vi "CCD spectrum processing_Shaowei-v5.vi"() -> ()   [LabVIEW 2012]
uses:
  <vilib>/Utility/file.llb/Read From Spreadsheet File (string).vi
  <vilib>/Utility/file.llb/Read From Spreadsheet File (DBL).vi
panel:
  out "Data Information":string[](array[string])
  in  "dI/dV Input Channel":i32=5
  out "File Information":string[][](array[string])
  out "Normalized dI/dV":cluster{"first row":dbl[], dbl[]}(graph)
  out "I":cluster{cluster{dbl, dbl}[]}[](graph)
  out "dI/dV":cluster{cluster{dbl, dbl}[]}[](graph)
  out "I":cluster{cluster{dbl, dbl}[]}[](graph)
  out "Spec1 File name 3":string
  out "Spec1 File name 2":string
  in  "select":bool
  in  "next":bool
  in  "previous":bool
  in  "Do it":bool
  out "?":path=path "F:/Bias-Spectroscopy113.dat"
  # "Input File"
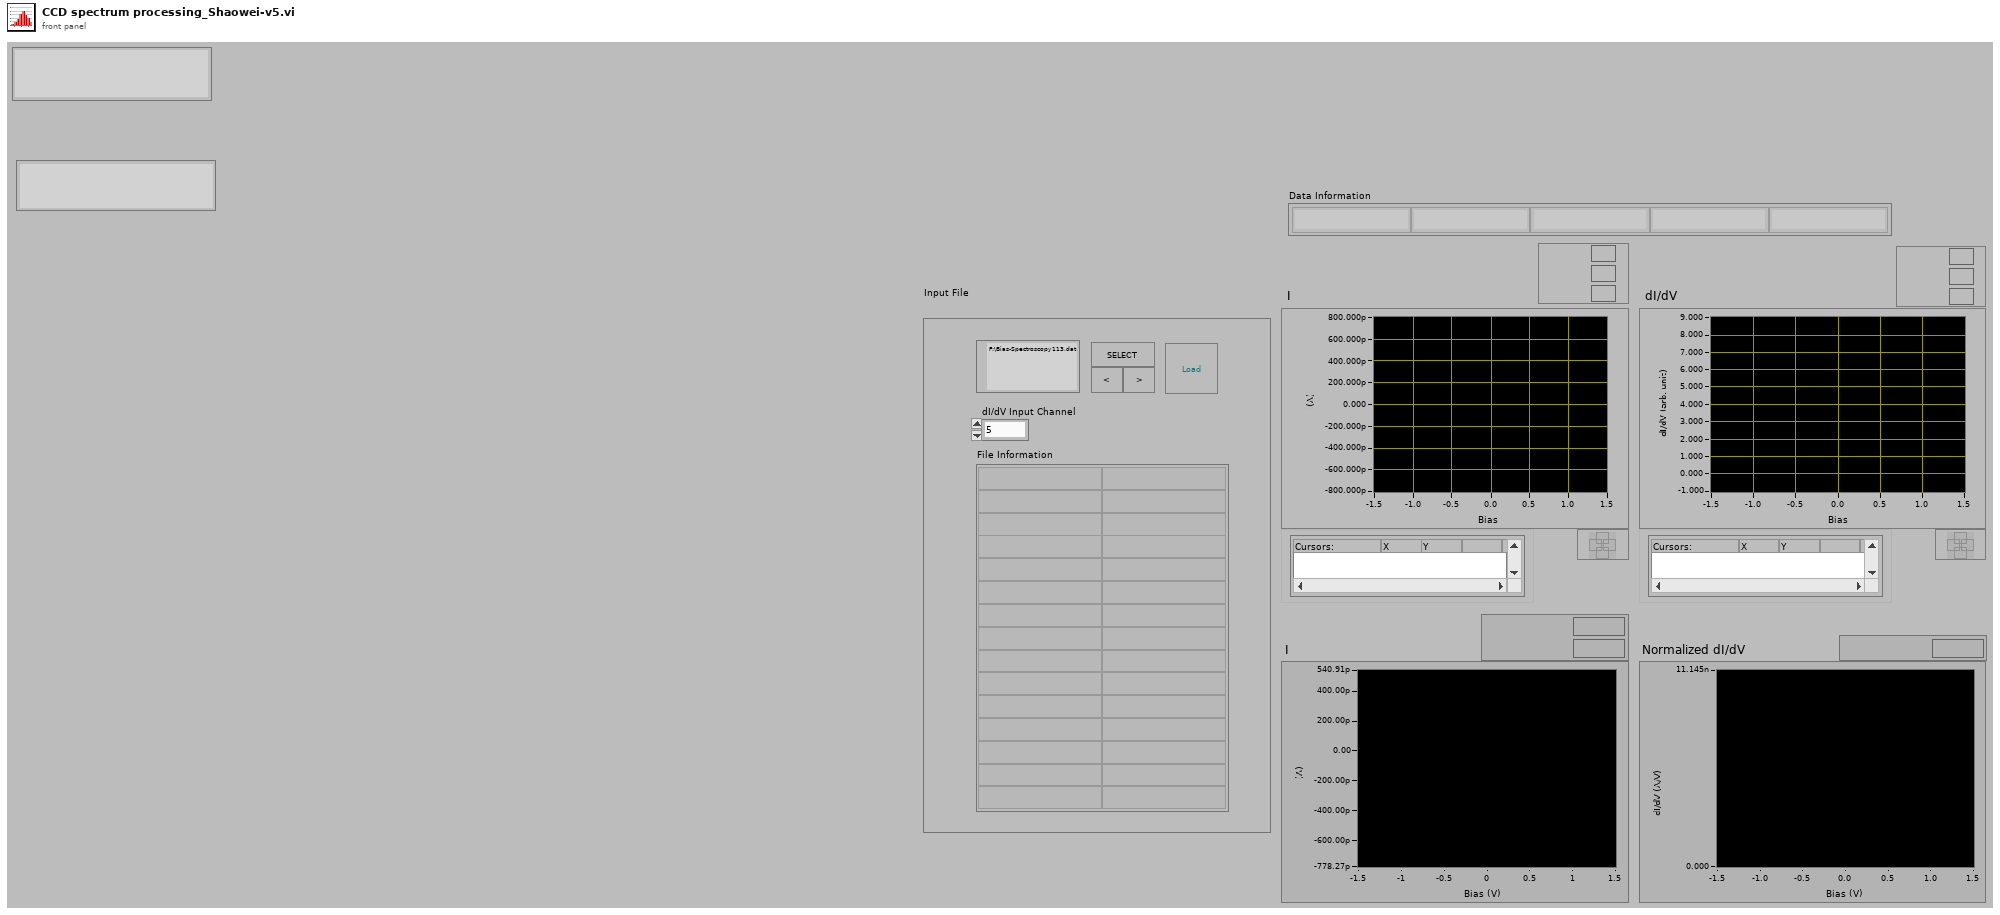
[diagram p1: front panel]
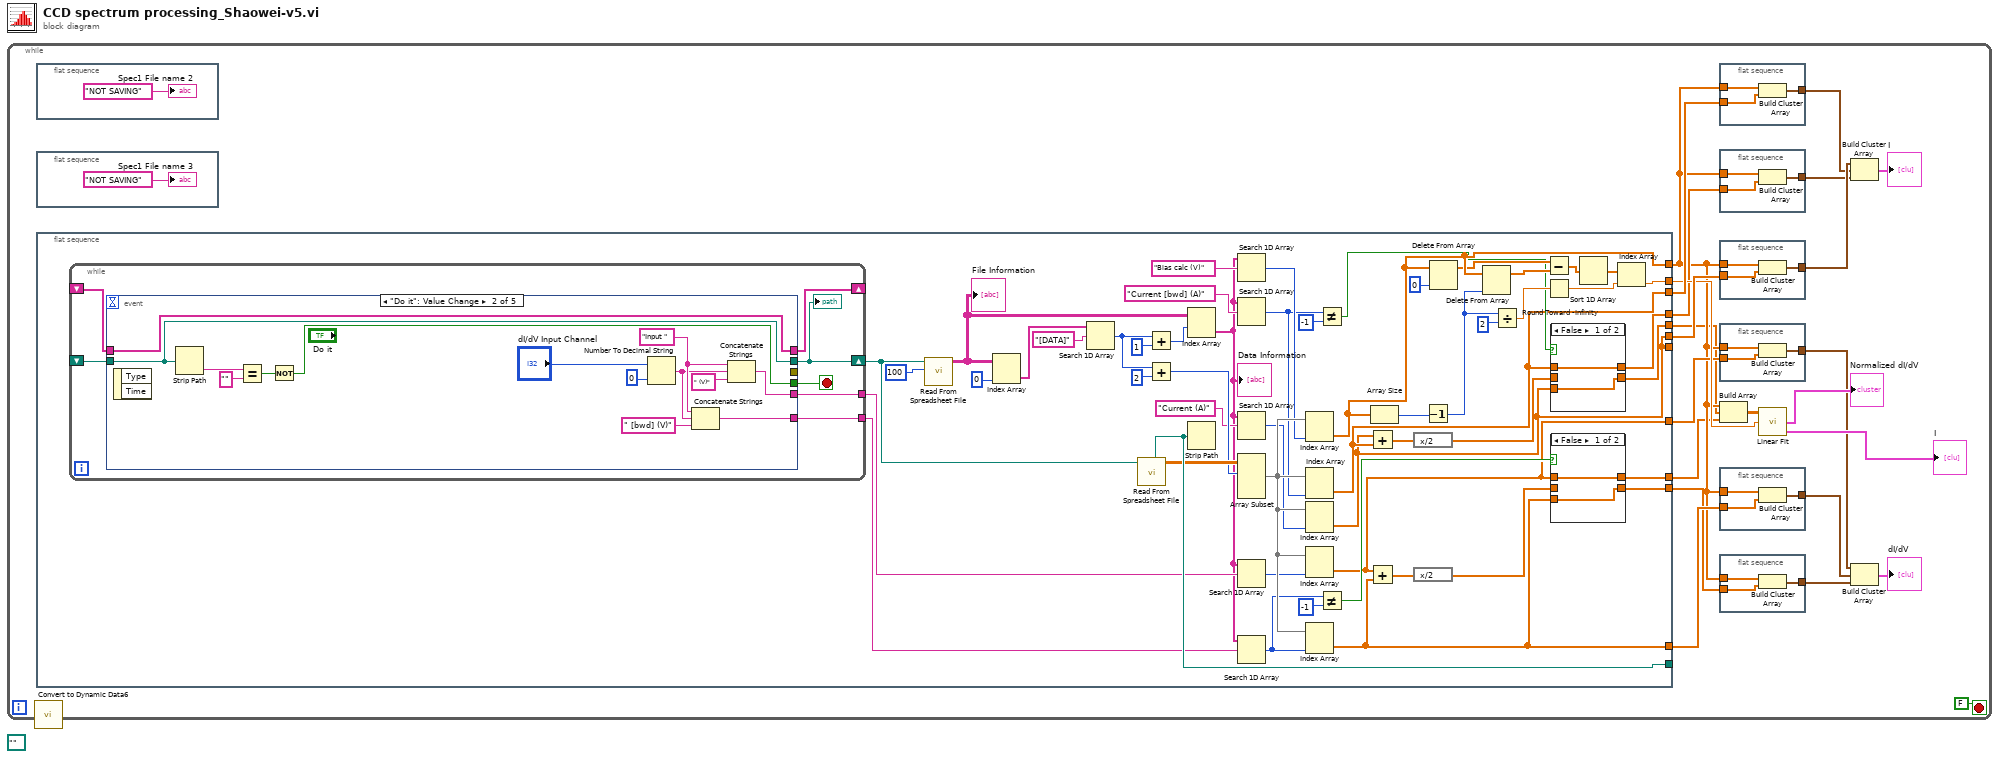
[diagram p0: block diagram]
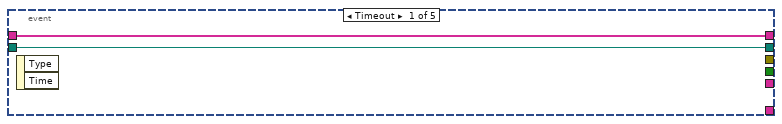
[diagram p4: hidden frame]
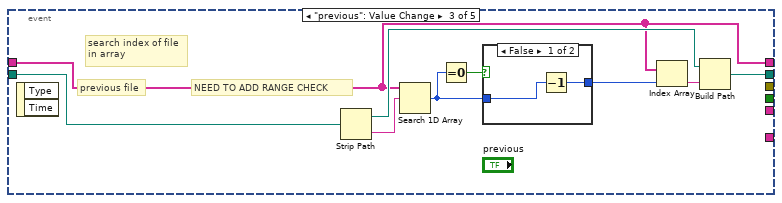
[diagram p5: hidden frame]
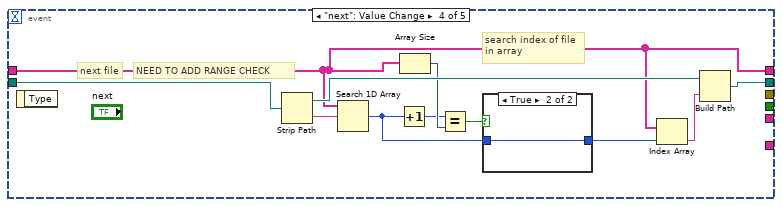
[diagram p7: hidden frame]
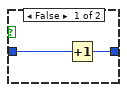
[diagram p8: hidden frame]
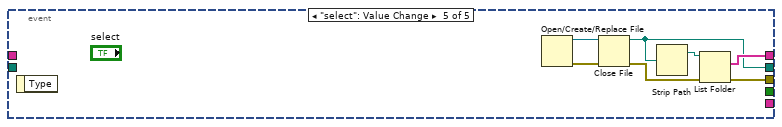
[diagram p9: hidden frame]
diagram:
  (unwired) path "" ("new file path (Not A Path if cancelled)")
  n1 = while {
    stop <- FALSE ("stop 2") stop-if-true
    n2 = call "Convert to Dynamic Data6"() -> ()  [unwired: 4 in, 1 out]
    n3 = flat-sequence {
      frame #0 {
        "Spec1 File name 2" <- "NOT SAVING"
      }
    }
    n4 = flat-sequence {
      frame #0 {
        "Spec1 File name 3" <- "NOT SAVING"
      }
    }
    n5 = flat-sequence {
      tunnel: [w92] -> _
      tunnel: [w89] -> w5
      tunnel: [w41] -> w21
      tunnel: [w45] -> w19
      tunnel: [w43] -> w14
      tunnel: [w44] -> w20
      tunnel: [w79] -> w17
      tunnel: [w41] -> _
      tunnel: [w53] -> w7
      tunnel: [w46] -> w4
      tunnel: [w42] -> w2
      tunnel: [w40] -> w1
      frame #0 {
        n6 = while {
          shift-right: [w104] -> _
          shift-left: _ -> [w103]
          shift-right: [w105] -> w78
          shift-left: _ -> [w102]
          tunnel: [w100] -> w63
          tunnel: [w99] -> w58
          stop <- w101 stop-if-true
          n7 = event shown="[1] \"Do it\": Value Change" {
            selector: _ -> [_ _ _ _ _]
            dyn-events: _ -> [_ _ _ _ _]
            timeout: _ -> [_ _ _ _ _]
            tunnel: [_ w117 _ _ _] -> w101
            tunnel: [w106 w120 w125 w141 w151] -> w105
            tunnel: [w107 w121 w127 w136 w152] -> w104
            tunnel: w103 -> [w107 w121 w127 w136 _]
            tunnel: w102 -> [w106 w120 w130 w140 _]
            tunnel: [_ _ _ _ w148] -> _
            tunnel: [_ w112 _ _ _] -> w100
            tunnel: [_ w108 _ _ _] -> w99
            event Timeout {
              n8 = event-data() -> ()  [unwired: 1 in, 2 out]
            }
            event "Do it": Value Change {
              w111 = "Input "
              n9 = event-data() -> ()  [unwired: 1 in, 2 out]
              n10 = Strip Path(path=w120) -> (name=w119:string)  [unwired: 1 out]
              n11 = Equal?(x=w119, y="") -> (x = y?=w116:bool)
              n12 = Not(x=w116) -> (.not. x?=w117:bool)
              n13 = Number To Decimal String(number="dI/dV Input Channel", width (-)=i16 0) -> (decimal integer string=w110:string)
              n14 = Concatenate Strings(w111, w110, " [bwd] (V)") -> (w108:string)
              n15 = Concatenate Strings(w111, w110, " (V)") -> (w112:string)
            }
            event "previous": Value Change {
              # "NEED TO ADD RANGE CHECK"
              # "previous file"
              # "search index of file\nin array"
              n16 = event-data() -> ()  [unwired: 1 in, 2 out]
              n17 = Strip Path(path=w130) -> (stripped path=w128:path, name=w129:string)
              n18 = Search 1D Array(1D array=w127, element=w129) -> (index of element=w123:i32)  [unwired: 1 in]
              n19 = Equal To 0?(x=w123) -> (x = 0?=w124:bool)
              n20 = case shown="False" w124 {
                tunnel: w123 -> [w132 w133]
                tunnel: [w131 w133] -> w122
                frame False {
                  n21 = Decrement(x=w132) -> (x-1=w131:i32)
                }
                frame True {
                }
              }
              n22 = Index Array(array=w127, index=w122) -> (element=w126:string)
              n23 = Build Path(base path=w128, name or relative path=w126) -> (appended path=w125:path)
            }
            event "next": Value Change {
              # "NEED TO ADD RANGE CHECK"
              # "next file"
              # "search index of file\nin array"
              n24 = event-data() -> ()  [unwired: 1 in, 1 out]
              n25 = Strip Path(path=w140) -> (stripped path=w143:path, name=w144:string)
              n26 = Search 1D Array(1D array=w136, element=w144) -> (index of element=w135:i32)  [unwired: 1 in]
              n27 = Increment(x=w135) -> (x+1=w137:i32)
              n28 = Array Size(array=w136) -> (size(s)=w139:i32)
              n29 = Equal?(x=w137, y=w139) -> (x = y?=w138:bool)
              n30 = case shown="True" w138 {
                tunnel: w135 -> [w146 w147]
                tunnel: [w145 w147] -> w134
                frame False {
                  n31 = Increment(x=w146) -> (x+1=w145:i32)
                }
                frame True {
                }
              }
              n32 = Index Array(array=w136, index=w134) -> (element=w142:string)
              n33 = Build Path(base path=w143, name or relative path=w142) -> (appended path=w141:path)
            }
            event "select": Value Change {
              n34 = event-data() -> ()  [unwired: 1 in, 1 out]
              n35 = Open/Create/Replace File() -> (refnum out=w154:refnum<file>, error out=w150:errorcluster)  [unwired: 6 in, 1 out]
              n36 = Close File(refnum=w154, error in=w150) -> (path=w151:path, error out=w149:errorcluster)
              n37 = Strip Path(path=w151) -> (stripped path=w153:path)  [unwired: 1 out]
              n38 = List Folder(path=w153, error in=w149) -> (filenames=w152:string[], error out=w148:errorcluster)  [unwired: 2 in, 2 out]
            }
          }
          "?" <- w105
        }
        n39 = call-poly <vilib>:"Read From Spreadsheet File.vi"("number of rows (all:-1)"=100, "file path (dialog if empty)"=w78) -> ("all rows"=w68:string[][])  [unwired: 5 in, 4 out]
        "File Information" <- w68
        n40 = Index Array(array=w68, index (col)=0 ("index")) -> (element=w74:string[])  [unwired: 1 in]
        n41 = Search 1D Array(1D array=w74, element="[DATA]") -> (index of element=w70:i32)  [unwired: 1 in]
        n42 = call-poly <vilib>:"Read From Spreadsheet File.vi"("file path (dialog if empty)"=w78) -> ("all rows"=w76:dbl[][], "new file path (Not A Path if cancelled)"=w92:path)  [unwired: 6 in, 3 out]
        n43 = Add(x=w70, y=1) -> (x+y=w67:i32)
        n44 = Add(x=w70, y=2) -> (x+y=w71:i32)
        n45 = Index Array(array=w68, index (row)=w67) -> (element=w59:string[])  [unwired: 1 in]
        "Data Information" <- w59
        n46 = Strip Path(path=w92) -> ()  [unwired: 2 out]
        n47 = Search 1D Array(1D array=w59, element="Bias calc (V)") -> (index of element=w65:i32)  [unwired: 1 in]
        n48 = Search 1D Array(1D array=w59, element="Current [bwd] (A)") -> (index of element=w56:i32)  [unwired: 1 in]
        n49 = Search 1D Array(1D array=w59, element="Current (A)") -> (index of element=w62:i32)  [unwired: 1 in]
        n50 = Array Subset(array=w76, index (row)=w71) -> (w91:dbl[][])  [unwired: 3 in]
        n51 = Search 1D Array(1D array=w59, element=w63) -> (index of element=w61:i32)  [unwired: 1 in]
        n52 = Search 1D Array(1D array=w59, element=w58) -> (index of element=w50:i32)  [unwired: 1 in]
        n53 = Index Array(array=w91, index (col)=w65) -> (element=w89:dbl[])  [unwired: 1 in]
        n54 = Index Array(array=w91, index (col)=w56) -> (element=w45:dbl[])  [unwired: 1 in]
        n55 = Index Array(array=w91, index (col)=w62) -> (element=w41:dbl[])  [unwired: 1 in]
        n56 = Index Array(array=w91, index (col)=w61) -> (element=w43:dbl[])  [unwired: 1 in]
        n57 = Index Array(array=w91, index (col)=w50) -> (element=w44:dbl[])  [unwired: 1 in]
        n58 = Not Equal?(x=w56, y=-1) -> (x != y?=w54:bool)
        n59 = Not Equal?(x=w50, y=-1) -> (x != y?=w49:bool)
        n60 = Add(x=w41, y=w45) -> (x+y=w57:dbl[])
        n61 = Add(x=w43, y=w44) -> (x+y=w48:dbl[])
        n62 = Array Size(array=w89) -> (size(s)=w88:i32)
        n63 = expression code="x/2"(w57) -> (w52:dbl[])
        n64 = expression code="x/2"(w48) -> (w47:dbl[])
        n65 = Decrement(x=w88) -> (x-1=w83:i32)
        n66 = Delete From Array(array=w89, index=0) -> (array with subset deleted=w86:dbl[])  [unwired: 1 in, 1 out]
        n67 = Delete From Array(array=w89, index=w83) -> (array with subset deleted=w87:dbl[])  [unwired: 1 in, 1 out]
        n68 = Divide(x=w83, y=2) -> (x/y=w81:dbl)
        n69 = Subtract(x=w86, y=w87) -> (x-y=w85:dbl[])
        n70 = Round Toward -Infinity(1:w81) -> (0:w80:dbl)
        n71 = case shown="False" w54 {
          tunnel: w52 -> [_ w98]
          tunnel: [w97 w98] -> w53
          tunnel: w45 -> [w97 _]
          tunnel: [w96 w98] -> w40
          tunnel: w41 -> [w96 _]
          frame False {
          }
          frame True {
          }
        }
        n72 = case shown="False" w49 {
          tunnel: w47 -> [_ w95]
          tunnel: [w94 w95] -> w46
          tunnel: w44 -> [w94 _]
          tunnel: [w93 w95] -> w42
          tunnel: w43 -> [w93 _]
          frame False {
          }
          frame True {
          }
        }
        n73 = Sort 1D Array(array=w85) -> (sorted array=w84:dbl[])
        n74 = Index Array(array=w84, index=w80) -> (element=w79:dbl)
      }
    }
    n75 = flat-sequence {
      tunnel: w5 -> [w34]
      tunnel: w19 -> [w33]
      tunnel: [w32] -> w9
      frame #0 {
        n76 = Build Cluster Array(w34, w33) -> (w32:cluster{dbl, dbl}[])
      }
    }
    n77 = flat-sequence {
      tunnel: w5 -> [w28]
      tunnel: w7 -> [w27]
      tunnel: [w26] -> w6
      frame #0 {
        n78 = Build Cluster Array(w28, w27) -> (w26:cluster{dbl, dbl}[])
      }
    }
    n79 = flat-sequence {
      tunnel: w5 -> [w157]
      tunnel: w21 -> [w156]
      tunnel: [w155] -> w10
      frame #0 {
        n80 = Build Cluster Array(w157, w156) -> (w155:cluster{dbl, dbl}[])
      }
    }
    n81 = flat-sequence {
      tunnel: w5 -> [w37]
      tunnel: w14 -> [w36]
      tunnel: [w35] -> w12
      frame #0 {
        n82 = Build Cluster Array(w37, w36) -> (w35:cluster{dbl, dbl}[])
      }
    }
    n83 = Build Array(w5, w1, w2) -> (w18:dbl[][])
    n84 = flat-sequence {
      tunnel: w5 -> [w31]
      tunnel: w20 -> [w30]
      tunnel: [w29] -> w13
      frame #0 {
        n85 = Build Cluster Array(w31, w30) -> (w29:cluster{dbl, dbl}[])
      }
    }
    n86 = flat-sequence {
      tunnel: w5 -> [w25]
      tunnel: w4 -> [w24]
      tunnel: [w23] -> w3
      frame #0 {
        n87 = Build Cluster Array(w25, w24) -> (w23:cluster{dbl, dbl}[])
      }
    }
    n88 = call "Linear Fit.vi"("Stepsize: V"=w17, "V, f, f'"=w18) -> ("Observed Data and Fitted Curve"=→"I":cluster{cluster{dbl, dbl}[]}[], "Calibrated Curve"=→"Normalized dI/dV":cluster{"first row":dbl[], dbl[]})  [unwired: 1 in, 1 out]
    n89 = Build Cluster Array(w10, w9, w6) -> (→"I":cluster{cluster{dbl, dbl}[]}[])
    n90 = Build Cluster Array(w12, w13, w3) -> (→"dI/dV":cluster{cluster{dbl, dbl}[]}[])
  }
